vi "GaGe4_QueryAcquisition .vi"(8 "error in (no error)":errorcluster, 11 "Handle Cluster in":T2) -> (0 "error out":errorcluster, 1 "Ext. clock":bool, 2 "Sample Rate":dbl, 3 "Output Handle Cluster":T1, 4 "Total points":i64, 5 "Mode":u16(ring)=1 items=["Single", "Dual", "Quad", "Octal"], 6 "Pre-trigger points":i64)   [LabVIEW 2015]
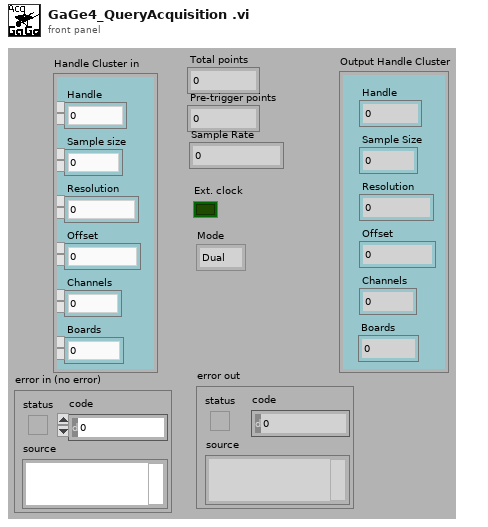
[diagram p1: front panel]
types:
  T1 = cluster{"Handle":u32, "Sample Size":u32, "Resolution":i32, "Offset":i32, "Channels":u32, "Boards":u32}
  T2 = cluster{"Handle":u32, "Sample size":u32, "Resolution":i32, "Offset":i32, "Channels":u32, "Boards":u32}
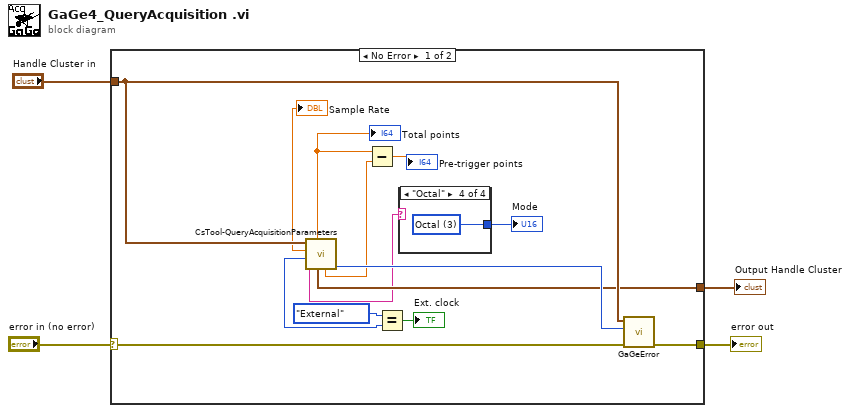
[diagram p0: block diagram]
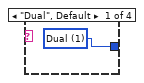
[diagram p2: hidden frame]
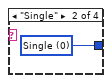
[diagram p3: hidden frame]
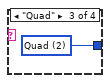
[diagram p4: hidden frame]
diagram:
  n1 = case shown="No Error" "error in (no error)" {
    selector: "error in (no error)" -> [w18 w24]
    tunnel: [w17 w24] -> w3
    tunnel: "Handle Cluster in" -> [w15 w23]
    tunnel: [w7 w23] -> w1
    frame No Error {
      n2 = call "CsTool-QueryAcquisitionParameters.vi"("Handle Cluster"=w15) -> ("Error Code"=w16:i32, "Depth"=w13:dbl, "Output Handle Cluster"=w7:T1, "Segment Size"=w14:dbl, "Mode"=w6:string, "Clock Mode"=w9:enum16{"Internal", "External", "Reference"}, "Sample Rate"=→"Sample Rate":dbl)  [unwired: 4 out]
      "Total points" <- w14
      n3 = Subtract(x=w14, y=w13) -> (x-y=→"Pre-trigger points":dbl)
      n4 = Equal?(x=enum16{"Internal", "External", "Reference"}."External" ("Clock Mode"), y=w9) -> (x = y?=→"Ext. clock":bool)
      n5 = case shown="\"Octal\"" w6 {
        tunnel: [w19 w20 w21 w22] -> w5
        frame "Dual", Default {
          w19 = u16 1 items=["Single", "Dual", "Quad", "Octal"] ("Mode")
        }
        frame "Single" {
          w20 = u16 0 items=["Single", "Dual", "Quad", "Octal"] ("Mode")
        }
        frame "Quad" {
          w21 = u16 2 items=["Single", "Dual", "Quad", "Octal"] ("Mode")
        }
        frame "Octal" {
          w22 = u16 3 items=["Single", "Dual", "Quad", "Octal"] ("Mode")
        }
      }
      "Mode" <- w5
      n6 = call "GaGeError.vi"("error in (no error)"=w18, "Error Code"=w16, "Handle Cluster"=w15) -> ("error out"=w17:errorcluster)  [unwired: 3 in, 5 out]
    }
    frame Error {
    }
  }
  "error out" <- w3
  "Output Handle Cluster" <- w1
